vi "Decimal to Degrees Minutes Seconds.vi"(11 "Lat Long Input (decimal)":dbl format="%#.7g") -> (1 "Seonds":dbl format="%#.5g", 2 "Minutes":dbl, 3 "Degrees":dbl)   [LabVIEW 2014]
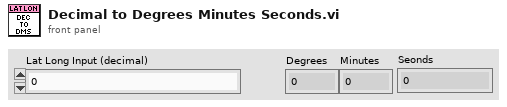
[diagram p1: front panel]
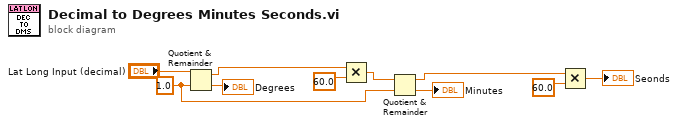
[diagram p0: block diagram]
diagram:
  w2 = 1.0 ("y")
  n1 = Quotient & Remainder(x="Lat Long Input (decimal)", y=w2) -> (x-y*floor(x/y)=w5:dbl, floor(x/y)=→"Degrees":dbl)
  n2 = Multiply(x=w5, y=60.0) -> (x*y=w9:dbl)
  n3 = Quotient & Remainder(x=w9, y=w2) -> (x-y*floor(x/y)=w3:dbl, floor(x/y)=→"Minutes":dbl)
  n4 = Multiply(x=w3, y=60.0) -> (x*y=→"Seonds":dbl)
